vi "Meas Panel.vi"(8 "error in":errorcluster, 11 "meas in":T1 {"swp cfg"."f list"."bias" format="%#_3p"; "swp cfg"."f list"."level" format="%#_3p"; "swp cfg"."f list"."fs [Hz]" format="%#_5p"; "swp cfg"."f list"."time [s]" format="%#_3p"; "swp cfg"."f list"."f/fs" format="%#_3p"; "swp cfg"."f list"."periods" format="%#_3f"; "swp cfg"."f list"."f [Hz]" format="%#_5p"}) -> (0 "error out":errorcluster, 2 "OK":bool, 3 "meas out":T1 {"swp cfg"."f list"."bias" format="%#_3p"; "swp cfg"."f list"."level" format="%#_3p"; "swp cfg"."f list"."fs [Hz]" format="%#_5p"; "swp cfg"."f list"."time [s]" format="%#_3p"; "swp cfg"."f list"."f/fs" format="%#_3p"; "swp cfg"."f list"."periods" format="%#_3f"; "swp cfg"."f list"."f [Hz]" format="%#_5p"})   [LabVIEW 2013]
uses:
  meas_swp_mode.ctl
  meas_sweep_flist_mode.ctl
  Meas Freq Info.ctl
  meas session.ctl
  Meas Sweep Config.ctl
  bridge/Bridge Session.ctl
  bridge/Bridge Type.ctl
  drivers/TWM client/TWM Session.ctl
  drivers/TWM client/TWM parameters.ctl
  source/Source Session.ctl
  source/Source Type.ctl
  drivers/AFG3101C/AFG3101C Session.ctl
  Meas Results.ctl
  bridge/Bridge Frequency Readings Data.ctl
  varilib/SGUI Assign References Mode.ctl
  varilib/varilib.lvlib
panel:
  in  "Tab Control 4":enum32{"Page 1", "Page 2"}(tab)
  out "meas path":path caption="Measurement path preview"
  in  "meas auto id":bool caption="Add auto-incremented index"
  in  "meas name":string caption="Measurement root name"
  in  "meas root":path caption="Measurement(s) root folder"
  in  "btn cancel":bool caption="OK Button"
  in  "Tab Control 3":enum32{"Page 1", "Page 2"}(tab)
  out "flist":T3[](array[typedef]) caption="Sweep list items" {"bias" format="%#_3p"; "level" format="%#_3p"; "fs [Hz]" format="%#_5p"; "time [s]" format="%#_3p"; "f/fs" format="%#_3p"; "periods" format="%#_3f"; "f [Hz]" format="%#_5p"}
  in  "btn ok":bool caption="OK Button"
  in  "Tab Control 2":enum32{"Page 1", "Page 2"}(tab)
  in  "subrec":i32=1 caption="Sub-records" min=1
  in  "Enable ALC?":bool
  in  "read delay [s]":dbl=1.0 caption="Readout extra delay [s]:" format="%#_6p"
  in  "Min settling [per]":dbl=1.0 caption="Min settling after level set [periods]:" format="%#_6p"
  in  "min settle [s]":dbl=1.0 caption="Min settling [s]:" format="%#_6p"
  in  "dc bias":dbl=5.0 caption="DC bias [A]" format="%#_6p"
  in  "adc fsf0 rat":dbl=4.0 caption="Min. fs/f0 ratio" min=0.0 format="%#_6p"
  in  "adc nper":dbl=5.0 caption="Min periods [-]" min=0.0 format="%#_6p"
  in  "t smpl":dbl=0.5 caption="Sampling time [s]" format="%#_6p"
  in  "Min fs [Hz]":dbl=50000.0 format="%#_6p"
  in  "level":dbl=5.0 caption="Source AC current [A]" format="%#_6p"
  in  "N":i32=5 caption="Samples per frequency" min=1
  in  "R":i32=1 caption="Samples to change frequency" min=1
  in  "avg":i32=1 caption="Averages" min=1
  in  "f0 coherent":bool caption="Coherent"
  in  "Tab Control":enum32{"Page 1", "Page 2"}(tab)
  in  "swp type":T4 caption="Mode"
  in  "freq swp rnd dig":dbl=50.0 caption="Rounding digits" min=0.0 format="%#_3f"
  in  "btn flst save":bool
  in  "btn flst load":bool
  in  "btn flst clr":bool
  in  "freq swp rnd":dbl=50.0 caption="Rounding [Hz]" min=0.0 format="%#_3p"
  in  "freq swp n":i32=1 caption="Sweep steps" min=1
  in  "swp mode":T5 caption="Sweep mode"
  in  "btn gen cust":bool
  in  "btn gen sgl":bool
  in  "btn gen step":bool
  in  "freq max":dbl=10000.0 caption="Stop frequency [Hz]" format="%#_6p"
  in  "freq min":dbl=50.0 caption="Start frequency [Hz]" format="%#_6p"
  in  "freq lst":dbl[](array[numeric]) caption="Frequency list [Hz]" format="%#_6p"
  in  "freq step":dbl=50.0 caption="Frequency step [Hz]" min=0.0 format="%#_6p"
  in  "freq sgl":dbl=1000.0 caption="Single frequency [Hz]" format="%#_6p"
  in  "rnd swp":bool caption="Random order"
  # "ADC setup"
  # "Timing"
  # "Sequencing"
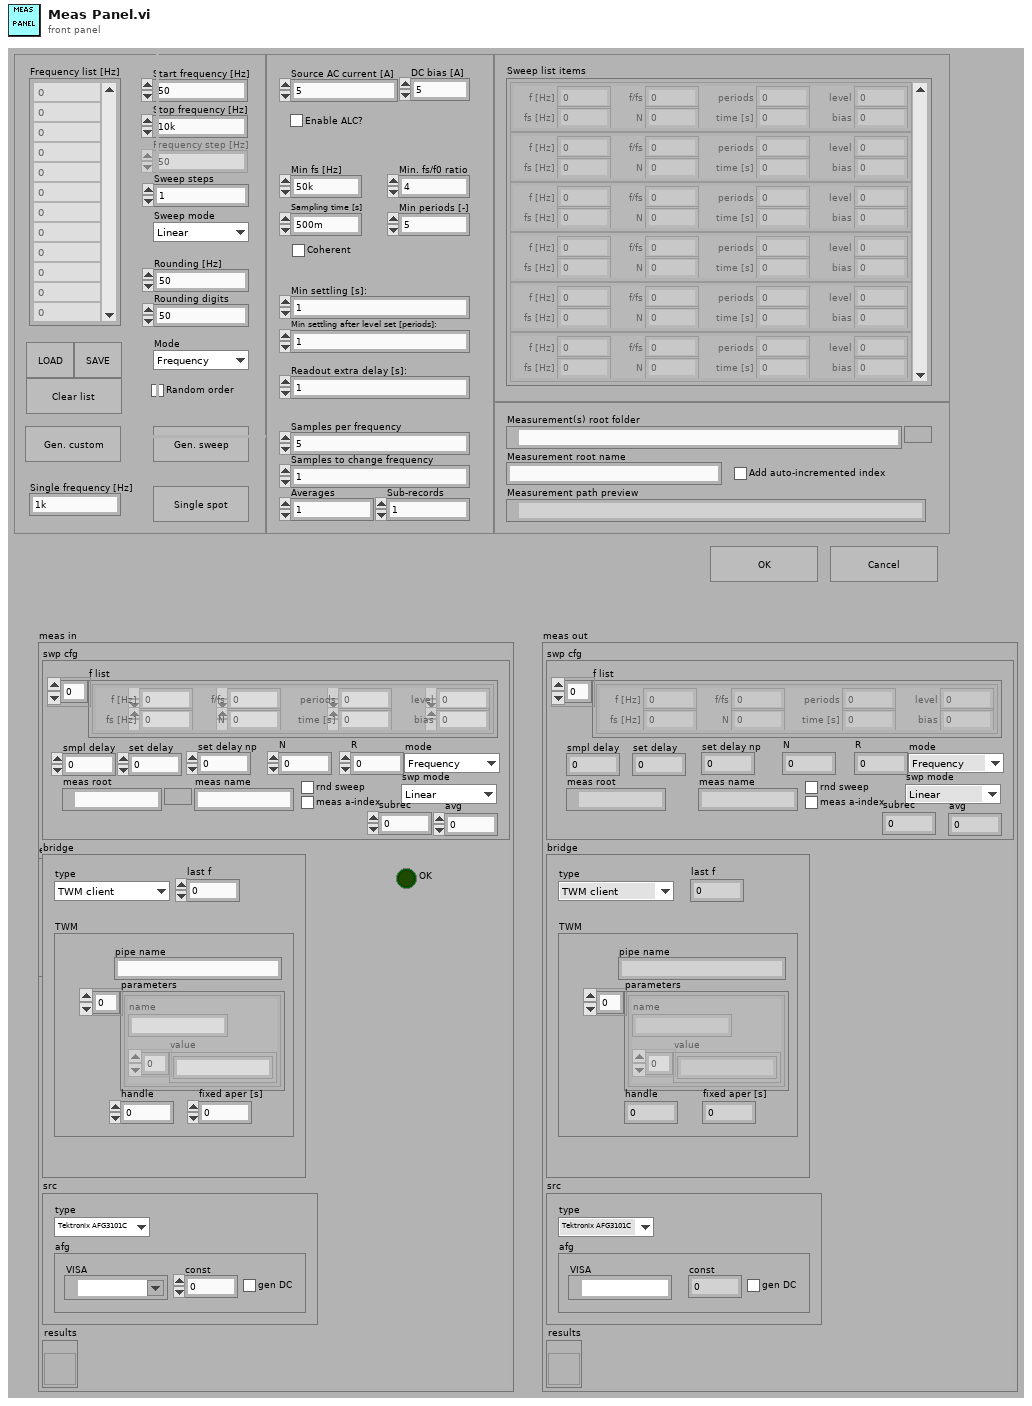
[diagram p1: front panel]
types:
  T1 = typedef "meas session.ctl" = cluster{"swp cfg":T2, "bridge":T6, "src":T10, "results":refnum<vi>}
  T2 = typedef "Meas Sweep Config.ctl" = cluster{"N":i32, "R":i32, "f list":T3[], "smpl delay":dbl, "set delay":dbl, "set delay np":dbl, "meas root":path, "meas name":string, "meas a-index":bool, "rnd sweep":bool, "mode":T4, "swp mode":T5, "avg":i32, "subrec":i32}
  T3 = typedef "Meas Freq Info.ctl" = cluster{"f [Hz]":dbl, "periods":dbl, "f/fs":dbl, "time [s]":dbl, "fs [Hz]":dbl, "N":i32, "level":dbl, "bias":dbl}
  T4 = typedef "meas_swp_mode.ctl" = enum16{"Frequency", "Level", "Bias"}
  T5 = typedef "meas_sweep_flist_mode.ctl" = enum16{"Linear", "Log10"}
  T6 = typedef "Bridge Session.ctl" = cluster{"type":T7, "TWM":T8, "last f":dbl}
  T7 = typedef "Bridge Type.ctl" = enum16{"TWM client", "dummy"}
  T8 = typedef "TWM Session.ctl" = cluster{"pipe name":string, "parameters":T9[], "handle":i32, "fixed aper [s]":dbl}
  T9 = typedef "TWM parameters.ctl" = cluster{"name":string, "value":string[]}
  T10 = typedef "Source Session.ctl" = cluster{"type":T11, "afg":T12}
  T11 = typedef "Source Type.ctl" = enum16{"Tektronix AFG3101C", "dummy"}
  T12 = typedef "AFG3101C Session.ctl" = cluster{"VISA":refnum<visa-resource-name>, "const":dbl, "gen DC":bool}
  T13 = typedef "varilib.lvlib/SGUI Assign References Mode.ctl" = enum16{"Add to stack", "Overwrite", "Release last", "Release ID"}
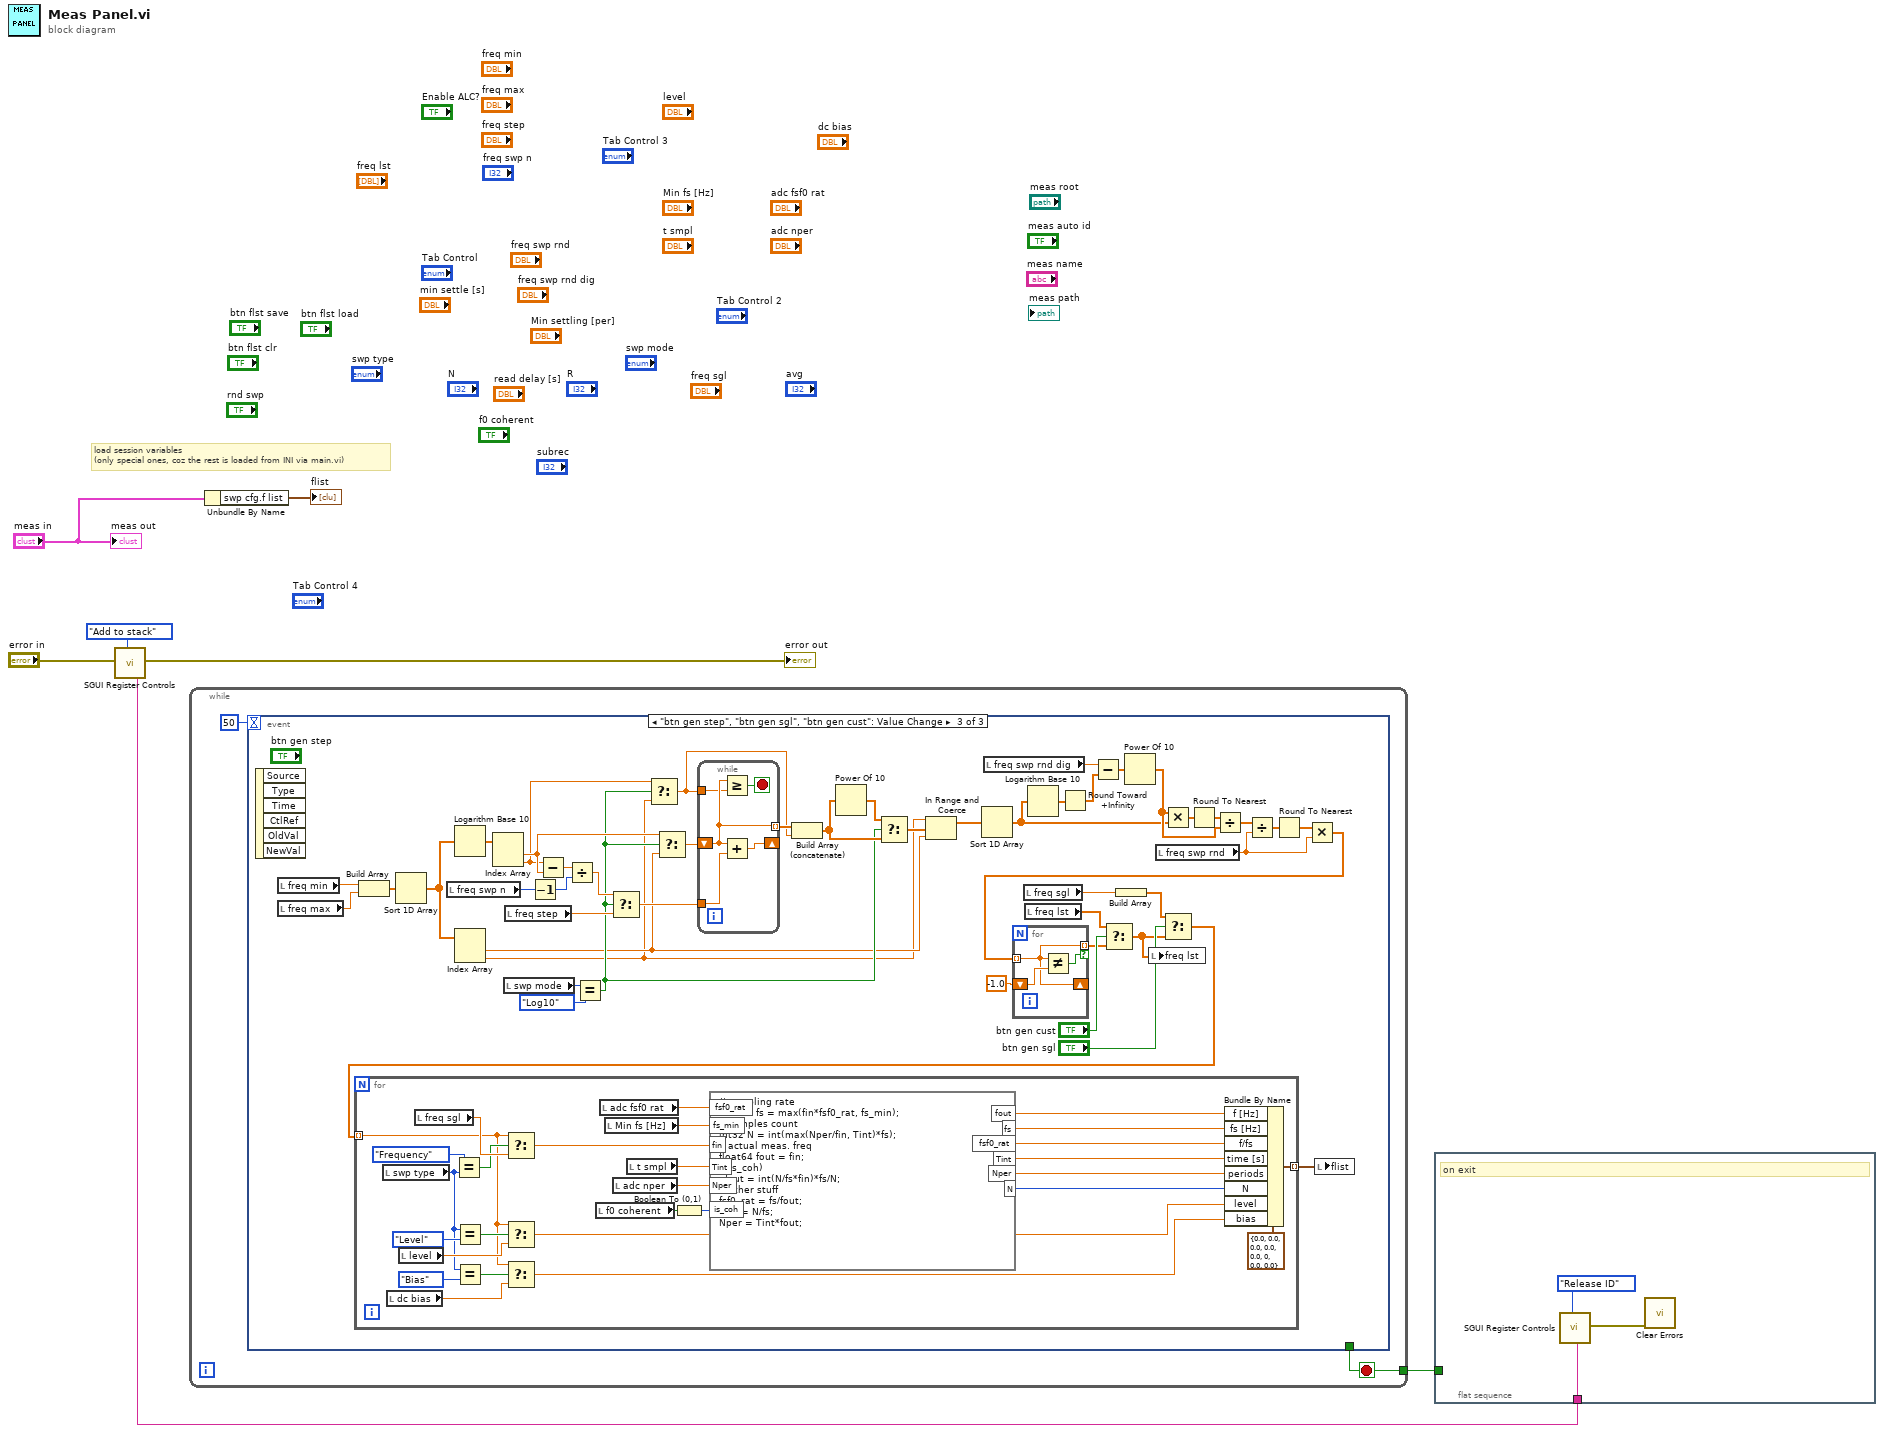
[diagram p0: block diagram]
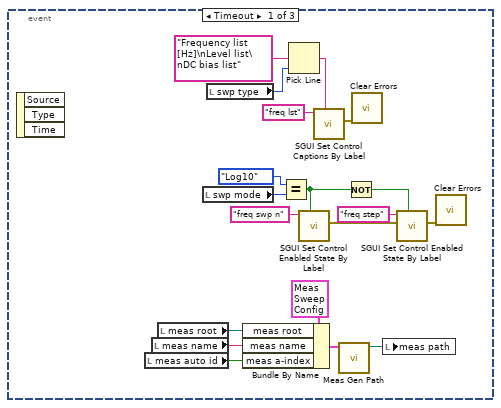
[diagram p2: hidden frame]
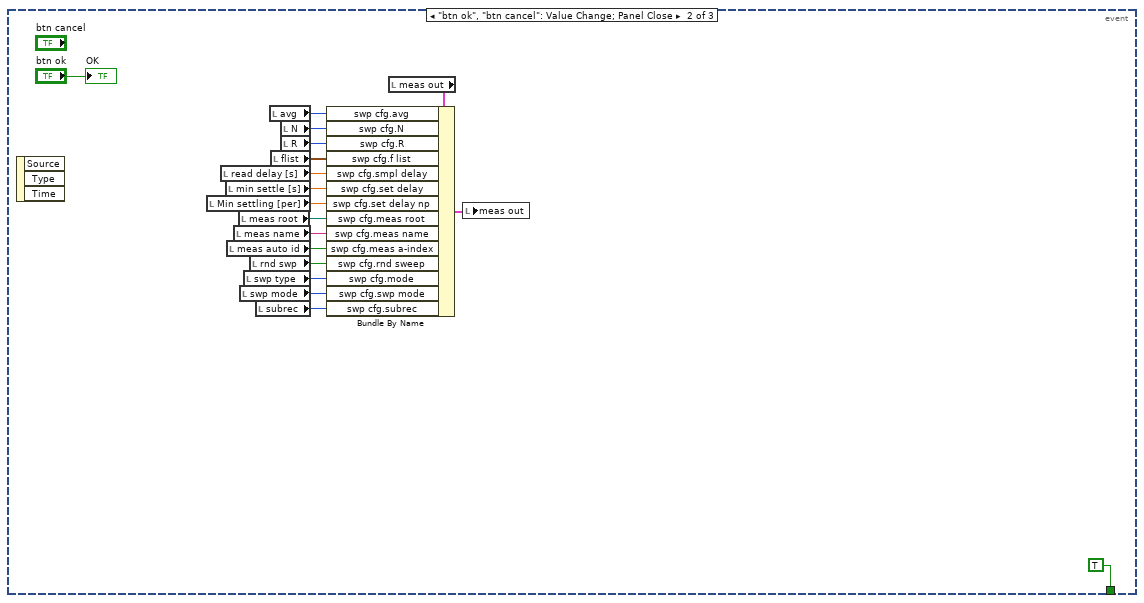
[diagram p3: hidden frame]
diagram:
  # "load session variables\n(only special ones, coz the rest is loaded from INI via main.vi)"
  n1 = call "SGUI Register Controls.vi"("error in"="error in", "register mode (overwrite)"=SGUI_Assign_References_Mode."Add to stack") -> ("assigned ID"=w5:string, "error out"=→"error out":errorcluster)  [unwired: 15 in, 1 out]
  n2 = while {
    tunnel: [w9] -> w6
    stop <- w9 stop-if-true
    n3 = event shown="[2] \"btn gen step\", \"btn gen sgl\", \"btn gen cust\": Value Change" {
      selector: _ -> [_ _ _]
      dyn-events: _ -> [_ _ _]
      timeout: 50 -> [_ _ _]
      tunnel: [_ TRUE _] -> w9
      event Timeout {
        n4 = event-data() -> ()  [unwired: 1 in, 3 out]
        n5 = local read "meas auto id"() -> (w11:bool)
        n6 = local read "meas name"() -> (w12:string)
        n7 = local read "meas root"() -> (w13:path)
        n8 = local read "swp mode"() -> (w24:T5)
        n9 = local read "swp type"() -> (w25:T4)
        n10 = Bundle By Name(cluster=T2 {"N"=0, "R"=0, "f list"=[], "smpl delay"=0.0, "set delay"=0.0, "set delay np"=0.0, "meas root"=path "", "meas name"="", "meas a-index"=FALSE, "rnd sweep"=FALSE, "mode"=enum."Frequency", "swp mode"=enum."Linear", "avg"=0, "subrec"=0} ("swp cfg"), "meas root"=w13, "meas name"=w12, "meas a-index"=w11) -> (w14:T2)
        n11 = Equal?(x=meas_sweep_flist_mode."Log10", y=w24) -> (x = y?=w19:bool)
        n12 = Pick Line(multi-line string="Frequency list [Hz]\nLevel list\nDC bias list", line index=w25) -> (output string=w26:string)  [unwired: 1 in]
        n13 = call "SGUI Set Control Enabled State By Label.vi"("labels (empty)"="freq swp n", "Enabled? (False)"=w19) -> ("error out"=w20:errorcluster)  [unwired: 8 in, 1 out]
        n14 = call "SGUI Set Control Captions By Label.vi"("labels (empty)"="freq lst", "captions (empty)"=w26) -> ("error out"=w17:errorcluster)  [unwired: 8 in, 1 out]
        n15 = call "Meas Gen Path.vi"("swp cfg"=w14) -> ("meas path"=w10:path)  [unwired: 10 in]
        n16 = Not(x=w19) -> (.not. x?=w18:bool)
        n17 = call <vilib>:"Clear Errors.vi"("error in (no error)"=w17) -> ()  [unwired: 6 in, 1 out]
        n18 = local write "meas path"(w10) -> ()
        n19 = call "SGUI Set Control Enabled State By Label.vi"("error in"=w20, "labels (empty)"="freq step", "Enabled? (False)"=w18) -> ("error out"=w16:errorcluster)  [unwired: 7 in, 1 out]
        n20 = call <vilib>:"Clear Errors.vi"("error in (no error)"=w16) -> ()  [unwired: 6 in, 1 out]
      }
      event "btn ok", "btn cancel": Value Change; Panel Close {
        n21 = event-data() -> ()  [unwired: 1 in, 3 out]
        n22 = local read "Min settling [per]"() -> (w38:dbl)
        n23 = local read "read delay [s]"() -> (w40:dbl)
        n24 = local read "min settle [s]"() -> (w39:dbl)
        n25 = local read "meas auto id"() -> (w35:bool)
        n26 = local read "meas name"() -> (w36:string)
        n27 = local read "meas root"() -> (w37:path)
        n28 = local read "swp mode"() -> (w31:T5)
        n29 = local read "swp type"() -> (w32:T4)
        n30 = local read "rnd swp"() -> (w34:bool)
        n31 = local read "subrec"() -> (w29:i32)
        n32 = local read "avg"() -> (w30:i32)
        n33 = local read "flist"() -> (w41:T3[])
        n34 = local read "N"() -> (w43:i32)
        n35 = local read "R"() -> (w42:i32)
        n36 = local read "meas out"() -> (w45:T1)
        n37 = Bundle By Name(cluster=w45, "swp cfg.avg"=w30, "swp cfg.N"=w43, "swp cfg.R"=w42, "swp cfg.f list"=w41, "swp cfg.smpl delay"=w40, "swp cfg.set delay"=w39, "swp cfg.set delay np"=w38, "swp cfg.meas root"=w37, "swp cfg.meas name"=w36, "swp cfg.meas a-index"=w35, "swp cfg.rnd sweep"=w34, "swp cfg.mode"=w32, "swp cfg.swp mode"=w31, "swp cfg.subrec"=w29) -> (w44:T1)
        n38 = local write "meas out"(w44) -> ()
        "OK" <- "btn ok"
      }
      event "btn gen step", "btn gen sgl", "btn gen cust": Value Change {
        n39 = event-data() -> ()  [unwired: 1 in, 6 out]
        n40 = local read "freq min"() -> (w94:dbl)
        n41 = local read "freq max"() -> (w93:dbl)
        n42 = Build Array(w94, w93) -> (w92:dbl[])
        n43 = Sort 1D Array(array=w92) -> (sorted array=w91:dbl[])
        n44 = local read "freq swp n"() -> (w88:i32)
        n45 = Logarithm Base 10(1:w91) -> (0:w90:dbl[])
        n46 = Index Array(array=w91) -> (element #1=w48:dbl, element #2=w47:dbl)  [unwired: 2 in]
        n47 = Index Array(array=w90) -> (element #1=w85:dbl, element #2=w83:dbl)  [unwired: 2 in]
        n48 = local read "swp mode"() -> (w76:T5)
        n49 = local read "freq step"() -> (w86:dbl)
        n50 = Decrement(x=w88) -> (x-1=w51:i32)
        n51 = Subtract(x=w83, y=w85) -> (x-y=w89:dbl)
        n52 = Divide(x=w89, y=w51) -> (x/y=w87:dbl)
        n53 = Equal?(x=w76, y=meas_sweep_flist_mode."Log10") -> (x = y?=w74:bool)
        n54 = Select(t=w87, s=w74, f=w86) -> (s? t:f=w84:dbl)
        n55 = Select(t=w83, s=w74, f=w47) -> (s? t:f=w78:dbl)
        n56 = Select(t=w85, s=w74, f=w48) -> (s? t:f=w81:dbl)
        n57 = while {
          tunnel: w84 -> [w130]
          tunnel: w78 -> [w127]
          shift-right: [w129] -> _
          shift-left: w81 -> [w128]
          tunnel: [w128] -> w82 mode=indexing
          stop <- w126 stop-if-true
          n58 = Greater Or Equal?(x=w128, y=w127) -> (x >= y?=w126:bool)
          n59 = Add(x=w128, y=w130) -> (x+y=w129:dbl)
        }
        n60 = Build Array (concatenate)(w82, w78) -> (w79:dbl[])
        n61 = Power Of 10(x=w79) -> (10^x=w80:dbl[])
        n62 = Select(t=w80, s=w74, f=w79) -> (s? t:f=w50:dbl[])
        n63 = In Range and Coerce(upper limit=w47, x=w50, lower limit=w48) -> (coerced(x)=w49:dbl[])  [unwired: 1 out]
        n64 = Sort 1D Array(array=w49) -> (sorted array=w66:dbl[])
        n65 = local read "freq swp rnd dig"() -> (w72:dbl)
        n66 = local read "freq sgl"() -> (w54:dbl)
        n67 = local read "freq lst"() -> (w57:dbl[])
        n68 = Logarithm Base 10(1:w66) -> (0:w73:dbl[])
        n69 = Round Toward +Infinity(x=w73) -> (ceil(x): smallest int >= x=w71:dbl[])
        n70 = Subtract(x=w72, y=w71) -> (x-y=w70:dbl[])
        n71 = Build Array(w54) -> (w55:dbl[])
        n72 = Power Of 10(x=w70) -> (10^x=w67:dbl[])
        n73 = local read "freq swp rnd"() -> (w62:dbl)
        n74 = Multiply(x=w67, y=w66) -> (x*y=w69:dbl[])
        n75 = Round To Nearest(number=w69) -> (nearest integer value=w68:dbl[])
        n76 = Divide(x=w68, y=w67) -> (x/y=w65:dbl[])
        n77 = Divide(x=w65, y=w62) -> (x/y=w64:dbl[])
        n78 = Round To Nearest(number=w64) -> (nearest integer value=w63:dbl[])
        n79 = Multiply(x=w63, y=w62) -> (x*y=w61:dbl[])
        n80 = for {
          tunnel: w61 -> [w124] mode=indexing
          shift-right: [w124] -> _
          shift-left: -1.0 -> [w125]
          tunnel: [w124] -> w59 mode=indexing if=w123
          n81 = Not Equal?(x=w124, y=w125) -> (x != y?=w123:bool)
        }
        n82 = Select(t=w57, s="btn gen cust", f=w59) -> (s? t:f=w56:dbl[])
        n83 = local write "freq lst"(w56) -> ()
        n84 = Select(t=w55, s="btn gen sgl", f=w56) -> (s? t:f=w53:dbl[])
        n85 = for {
          tunnel: w53 -> [w110] mode=indexing
          tunnel: [w121] -> w52 mode=indexing
          n86 = local read "swp type"() -> (w111:T4)
          n87 = local read "dc bias"() -> (w108:dbl)
          n88 = local read "level"() -> (w114:dbl)
          n89 = local read "freq sgl"() -> (w119:dbl)
          n90 = Equal?(x=meas_swp_mode."Frequency", y=w111) -> (x = y?=w117:bool)
          n91 = Equal?(x=w111, y=meas_swp_mode."Level") -> (x = y?=w115:bool)
          n92 = Equal?(x=w111, y=meas_swp_mode."Bias") -> (x = y?=w113:bool)
          n93 = Select(t=w110, s=w117, f=w119) -> (s? t:f=w106:dbl)
          n94 = Select(t=w110, s=w115, f=w114) -> (s? t:f=w118:dbl)
          n95 = Select(t=w110, s=w113, f=w108) -> (s? t:f=w109:dbl)
          n96 = local read "f0 coherent"() -> (w102:bool)
          n97 = local read "adc fsf0 rat"() -> (w107:dbl)
          n98 = local read "Min fs [Hz]"() -> (w105:dbl)
          n99 = local read "adc nper"() -> (w103:dbl)
          n100 = local read "t smpl"() -> (w104:dbl)
          n101 = Boolean To (0,1)(Boolean=w102) -> (0, 1=w101:i16)
          n102 = formula code="// sampling rate\nfloat64 fs = max(fin*fsf0_rat, fs_min);\n// samples count\nint32 N = int(max(Nper/fin, Tint)*fs);\n// actual meas. freq\nfloat64 fout = fin;\nif(is_coh)\n  fout = int(N/fs*fin)*fs/N;\n// other stuff\nfsf0_rat = fs/fout;\nTint = N/fs;\nNper = Tint*fout;"("fsf0_rat"=w107, "fs_min"=w105, "Tint"=w104, "Nper"=w103, "fin"=w106, "is_coh"=w101) -> ("fout"=w100:dbl, "fs"=w99:dbl, "Tint"=w97:dbl, "Nper"=w96:dbl, "fsf0_rat"=w98:dbl, "N"=w95:i32)
          n103 = Bundle By Name(cluster=T3 {"f [Hz]"=0.0, "periods"=0.0, "f/fs"=0.0, "time [s]"=0.0, "fs [Hz]"=0.0, "N"=0, "level"=0.0, "bias"=0.0} ("Cluster"), "f [Hz]"=w100, "fs [Hz]"=w99, "f/fs"=w98, "time [s]"=w97, "periods"=w96, "N"=w95, "level"=w118, "bias"=w109) -> (w121:T3)
        }
        n104 = local write "flist"(w52) -> ()
      }
    }
  }
  n105 = Unbundle By Name("meas in") -> ("swp cfg.f list"=→"flist":T3[])
  n106 = flat-sequence {
    tunnel: w6 -> [_]
    tunnel: w5 -> [w131]
    frame #0 {
      # "on exit"
      n107 = call "SGUI Register Controls.vi"("register mode (overwrite)"=SGUI_Assign_References_Mode."Release ID", "controls ID (empty)"=w131) -> ("error out"=w132:errorcluster)  [unwired: 15 in, 2 out]
      n108 = call <vilib>:"Clear Errors.vi"("error in (no error)"=w132) -> ()  [unwired: 6 in, 1 out]
    }
  }
  "meas out" <- "meas in"
